vi "CRYUpdate Repeat State Lib.vi"(0 "Start Index":i32, 1 "sOption":string, 5 "End Index":i32, 7 "Start":dbl format="%#_5g", 9 "Increment":dbl, 11 "Num":i32, 12 "Count":i32) -> ()   [LabVIEW 2013]
uses:
  CRYProject Editor Global.vi
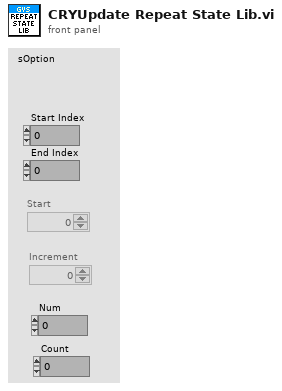
[diagram p1: front panel]
types:
  T1 = cluster{"Start":dbl, "Increment":dbl, "Count":i32, "Num":i32}
  T2 = typedef "CRYTS.ctl" = cluster{"No.TS":u16, "TS File Path":path, "TS Name":string, "EditStepName":string, "Steps":T3[], "New State":bool, "Change State":bool, "Flattened CurveLib Data":string, "Document Data":string, "EditStepNo":u16, "Operator Start File":string, "Sequence Type":string, "Sequence Language":string}
  T3 = typedef "CRYStep.ctl" = cluster{"No.VI":i32, "Category":string, "StepName":string, "Seq setup flattened":string, "Comment":string, "Steps config.":bool[], "Jump config":i32[], "Start":dbl, "Increment":dbl, "Name":string, "Unit":string, "Y data":u16, "Y prefix":string, "Y dB ref":dbl, "Y unit":string, "Repeat State Array":cluster{"Start":dbl, "Increment":dbl, "Count":i32, "Num":i32}[]}
  T4 = cluster{"Start":dbl, "Increment":dbl, "Count":i32, "Num":i32}[]
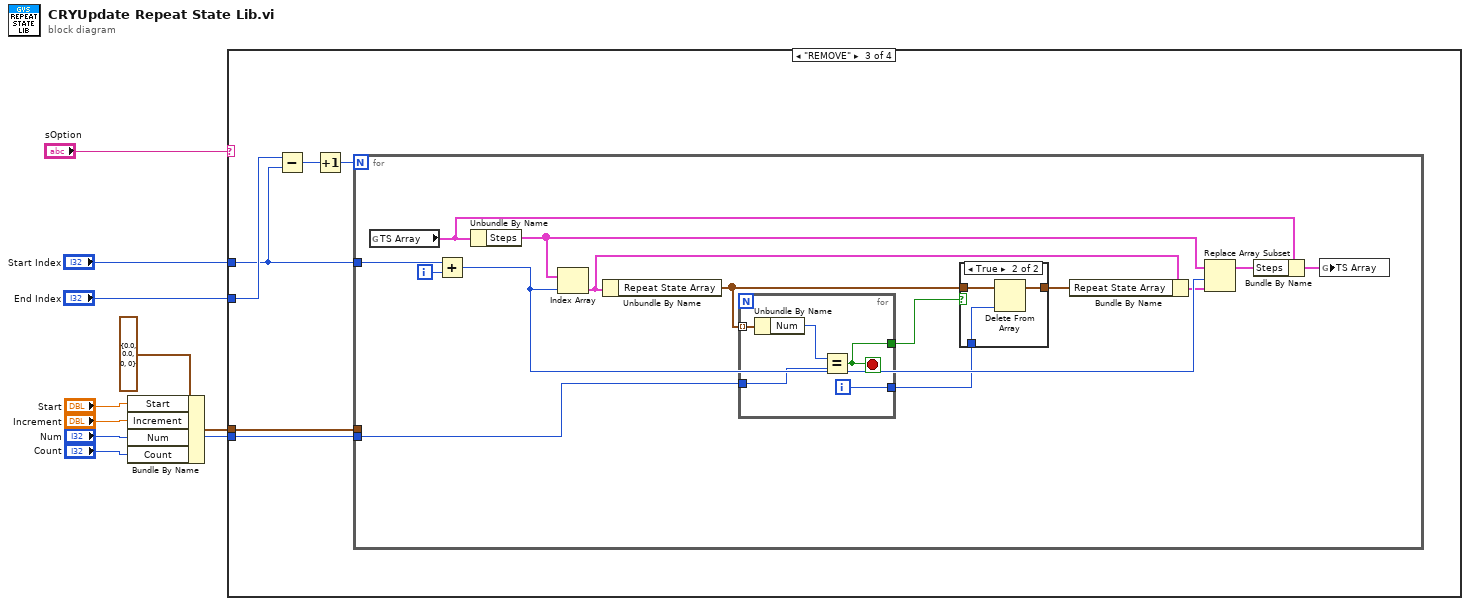
[diagram p0: block diagram]
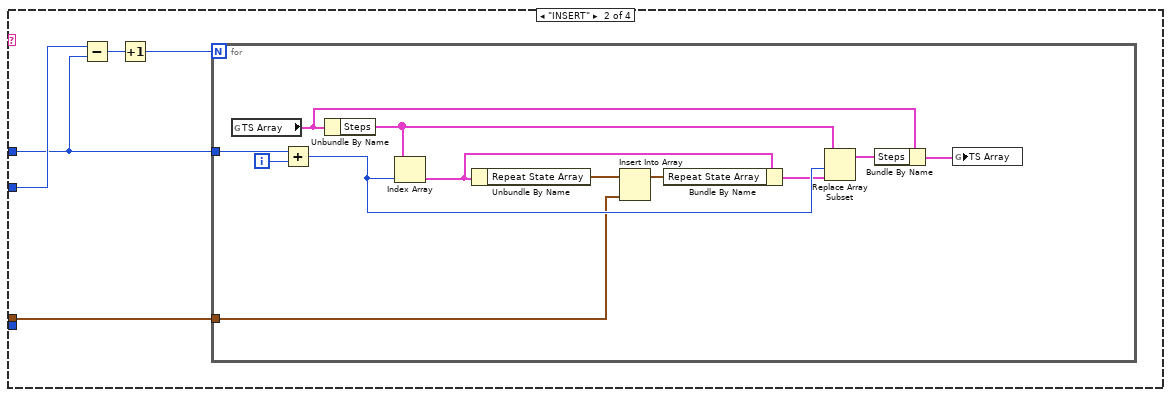
[diagram p3: hidden frame]
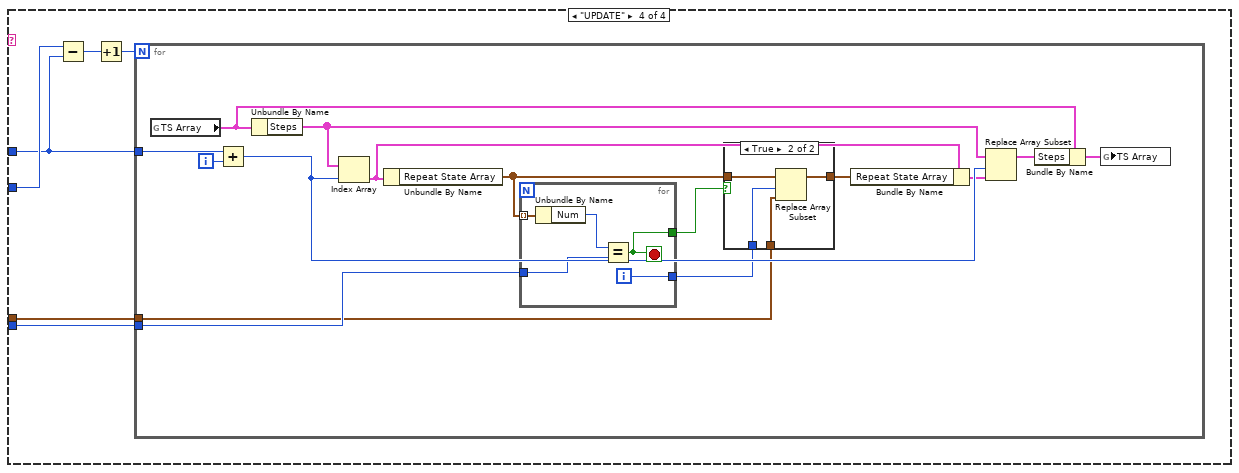
[diagram p5: hidden frame]
diagram:
  n1 = Bundle By Name(cluster=T1 {"Start"=0.0, "Increment"=0.0, "Count"=0, "Num"=0} ("new element/subarray"), "Start"="Start", "Increment"="Increment", "Num"="Num", "Count"="Count") -> (w2:T1)
  n2 = case shown="\"REMOVE\"" "sOption" {
    tunnel: "End Index" -> [_ w12 w30 w59]
    tunnel: "Start Index" -> [_ w11 w29 w58]
    tunnel: w2 -> [_ w10 w28 w57]
    tunnel: "Num" -> [_ _ w27 w56]
    frame Default {
    }
    frame "INSERT" {
      n3 = Subtract(x=w12, y=w11) -> (x-y=w14:i32)
      n4 = Increment(x=w14) -> (x+1=w13:i32)
      n5 = for {
        N: w13 -> [_]
        tunnel: w11 -> [w26]
        tunnel: w10 -> [w15]
        i -> [w25]
        n6 = global read "CRYProject Editor Global.vi" "TS Array"() -> (w18:T2)
        n7 = Add(x=w26, y=w25) -> (x+y=w21:i32)
        n8 = Unbundle By Name(w18) -> ("Steps"=w19:T3[])
        n9 = Index Array(array=w19, index=w21) -> (element=w23:T3)
        n10 = Unbundle By Name(w23) -> ("Repeat State Array"=w24:T4)
        n11 = Insert Into Array(array=w24, new element=w15) -> (w22:T4)  [unwired: 1 in]
        n12 = Bundle By Name(cluster=w23, "Repeat State Array"=w22) -> (w20:T3)
        n13 = Replace Array Subset(array=w19, new element=w20, index=w21) -> (w17:T3[])
        n14 = Bundle By Name(cluster=w18, "Steps"=w17) -> (w16:T2)
        n15 = global write "CRYProject Editor Global.vi" "TS Array"(w16) -> ()
      }
    }
    frame "REMOVE" {
      n16 = Subtract(x=w30, y=w29) -> (x-y=w32:i32)
      n17 = Increment(x=w32) -> (x+1=w31:i32)
      n18 = for {
        N: w31 -> [_]
        tunnel: w29 -> [w46]
        tunnel: w28 -> [_]
        tunnel: w27 -> [w35]
        i -> [w45]
        n19 = global read "CRYProject Editor Global.vi" "TS Array"() -> (w39:T2)
        n20 = Add(x=w46, y=w45) -> (x+y=w42:i32)
        n21 = Unbundle By Name(w39) -> ("Steps"=w40:T3[])
        n22 = Index Array(array=w40, index=w42) -> (element=w44:T3)
        n23 = Unbundle By Name(w44) -> ("Repeat State Array"=w36:T4)
        n24 = for {
          tunnel: w36 -> [w55] mode=indexing
          tunnel: w35 -> [w53]
          tunnel: [w52] -> w34
          tunnel: [w51] -> w33
          i -> [w52]
          stop <- w51 stop-if-true
          n25 = Unbundle By Name(w55) -> ("Num"=w54:i32)
          n26 = Equal?(x=w54, y=w53) -> (x = y?=w51:bool)
        }
        n27 = case shown="True" w33 {
          tunnel: [w47 w50] -> w43
          tunnel: w36 -> [w47 w49]
          tunnel: w34 -> [_ w48]
          frame False {
          }
          frame True {
            n28 = Delete From Array(array=w49, index=w48) -> (array with subset deleted=w50:T4)  [unwired: 1 in, 1 out]
          }
        }
        n29 = Bundle By Name(cluster=w44, "Repeat State Array"=w43) -> (w41:T3)
        n30 = Replace Array Subset(array=w40, new element=w41, index=w42) -> (w38:T3[])
        n31 = Bundle By Name(cluster=w39, "Steps"=w38) -> (w37:T2)
        n32 = global write "CRYProject Editor Global.vi" "TS Array"(w37) -> ()
      }
    }
    frame "UPDATE" {
      n33 = Subtract(x=w59, y=w58) -> (x-y=w61:i32)
      n34 = Increment(x=w61) -> (x+1=w60:i32)
      n35 = for {
        N: w60 -> [_]
        tunnel: w58 -> [w76]
        tunnel: w57 -> [w62]
        tunnel: w56 -> [w65]
        i -> [w75]
        n36 = global read "CRYProject Editor Global.vi" "TS Array"() -> (w69:T2)
        n37 = Add(x=w76, y=w75) -> (x+y=w72:i32)
        n38 = Unbundle By Name(w69) -> ("Steps"=w70:T3[])
        n39 = Index Array(array=w70, index=w72) -> (element=w74:T3)
        n40 = Unbundle By Name(w74) -> ("Repeat State Array"=w66:T4)
        n41 = for {
          tunnel: w66 -> [w86] mode=indexing
          tunnel: w65 -> [w84]
          tunnel: [w83] -> w64
          tunnel: [w82] -> w63
          i -> [w83]
          stop <- w82 stop-if-true
          n42 = Unbundle By Name(w86) -> ("Num"=w85:i32)
          n43 = Equal?(x=w85, y=w84) -> (x = y?=w82:bool)
        }
        n44 = case shown="True" w63 {
          tunnel: [w77 w81] -> w73
          tunnel: w66 -> [w77 w80]
          tunnel: w64 -> [_ w79]
          tunnel: w62 -> [_ w78]
          frame False {
          }
          frame True {
            n45 = Replace Array Subset(array=w80, new element=w78, index=w79) -> (w81:T4)
          }
        }
        n46 = Bundle By Name(cluster=w74, "Repeat State Array"=w73) -> (w71:T3)
        n47 = Replace Array Subset(array=w70, new element=w71, index=w72) -> (w68:T3[])
        n48 = Bundle By Name(cluster=w69, "Steps"=w68) -> (w67:T2)
        n49 = global write "CRYProject Editor Global.vi" "TS Array"(w67) -> ()
      }
    }
  }
